vi "convertTheRest.vi"(11 "byte [0, 1]":string) -> (1 "maxSpeed":string, 2 "negative incline":dbl, 3 "double precision float":dbl)   [LabVIEW 2018]
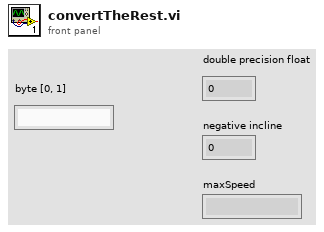
[diagram p1: front panel]
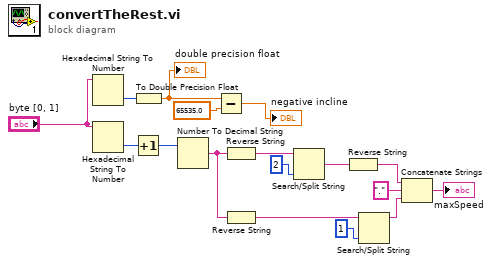
[diagram p0: block diagram]
diagram:
  n1 = Hexadecimal String To Number(string="byte [0, 1]") -> (number=w14:u32)  [unwired: 2 in, 1 out]
  n2 = Hexadecimal String To Number(string="byte [0, 1]") -> (number=w7:u32)  [unwired: 2 in, 1 out]
  n3 = Increment(x=w7) -> (x+1=w8:u32)
  n4 = To Double Precision Float(number=w14) -> (double precision float=w15:dbl)
  "double precision float" <- w15
  n5 = Number To Decimal String(number=w8) -> (decimal integer string=w6:string)  [unwired: 1 in]
  n6 = Subtract(x=w15, y=65535.0) -> (x-y=→"negative incline":dbl)
  n7 = Reverse String(1:w6) -> (0:w11:string)
  n8 = Reverse String(1:w6) -> (0:w10:string)
  n9 = Search/Split String(string=w11, offset (0)=2) -> (match + rest of string=w9:string)  [unwired: 1 in, 2 out]
  n10 = Reverse String(1:w9) -> (0:w12:string)
  n11 = Search/Split String(string=w10, offset (0)=1) -> (substring before match=w4:string)  [unwired: 1 in, 2 out]
  n12 = Concatenate Strings(w12, ".", w4) -> (→"maxSpeed":string)
